vi "CompareBoolArray.vi"(10 "dest in":bool[](array[boolean]), 11 "src in":bool[](array[boolean])) -> (2 "dest out":bool[](array[boolean]), 3 "equal":bool)   [LabVIEW 2018]
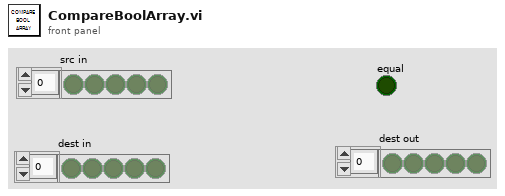
[diagram p1: front panel]
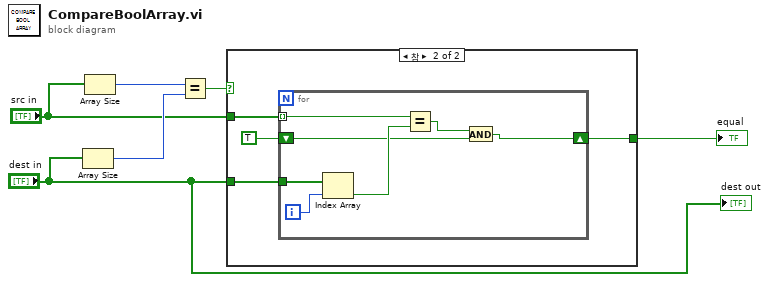
[diagram p0: block diagram]
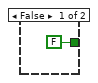
[diagram p2: hidden frame]
diagram:
  n1 = Array Size(array="dest in") -> (size(s)=w5:i32)
  n2 = Array Size(array="src in") -> (size(s)=w6:i32)
  n3 = Equal?(x=w6, y=w5) -> (x = y?=w3:bool)
  n4 = case shown="참" w3 {
    tunnel: "src in" -> [_ w11]
    tunnel: "dest in" -> [_ w10]
    tunnel: [FALSE w8] -> w2
    frame False {
    }
    frame True {
      n5 = for {
        tunnel: w11 -> [w16] mode=indexing
        tunnel: w10 -> [w18]
        shift-right: [w12] -> w8
        shift-left: TRUE -> [w13]
        i -> [w17]
        n6 = Index Array(array=w18, index=w17) -> (element=w15:bool)
        n7 = Equal?(x=w16, y=w15) -> (x = y?=w14:bool)
        n8 = And(x=w14, y=w13) -> (x .and. y?=w12:bool)
      }
    }
  }
  "equal" <- w2
  "dest out" <- "dest in"
